vi "System Mixed Checkbox.vi"() -> ()   [LabVIEW 2023]
doc: "Demonstrates how to use the system mixed checkbox."
panel:
  in  "Fail":string="Fail"
  in  "Pass":string="Pass"
  in  "Stop":bool
  in  "Test Result":enum8{"False", "True", "Mixed"}(c332)
  in  "Result List":i32[](listbox)
  # "Overview: Demonstrates the use of the System Mixed Checkbox control.\nInstructions:\n1. Run the VI.\n2. Select an item in the list, and notice its 'Result' value is reflected in the Passed? checkbox.\n3. Select multiple items in the list by Ctrl-clicking on them. If you selected any items with different 'Result' values, the Passed? checkbox will be in a mixed state.\n4. Change the Passed? checkbox value to apply the value to the selected list items.\n5. Click Stop to stop the VI."
  # "For this example, the Allow Mixed option in the System Mixed Checkbox right-click menu is deselected so the user cannot interactively set the checkbox value to a mixed state."
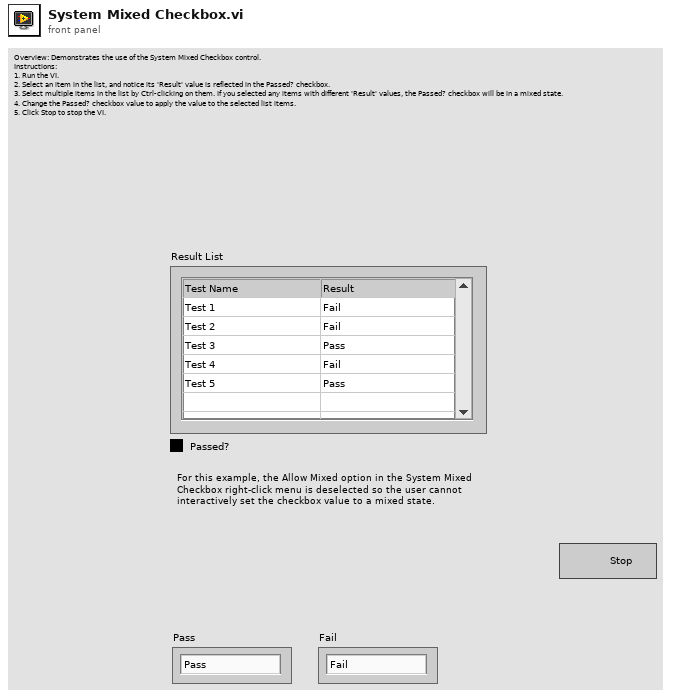
[diagram p1: front panel]
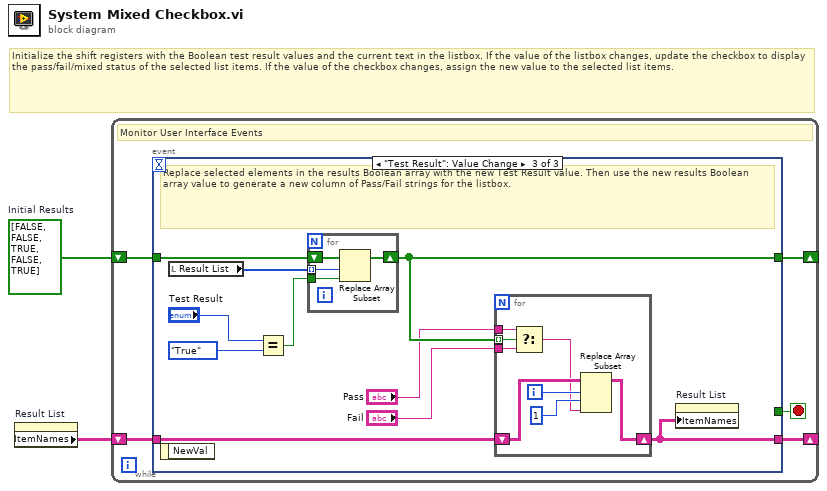
[diagram p0: block diagram]
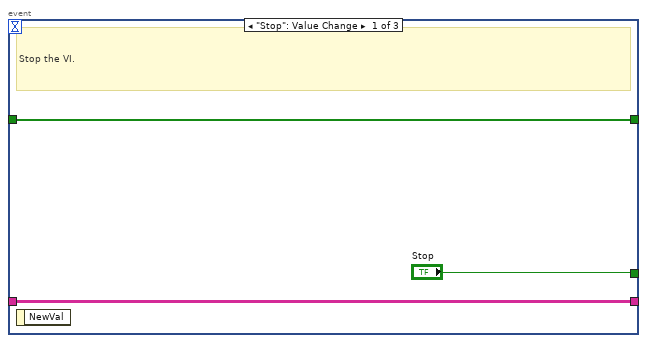
[diagram p2: hidden frame]
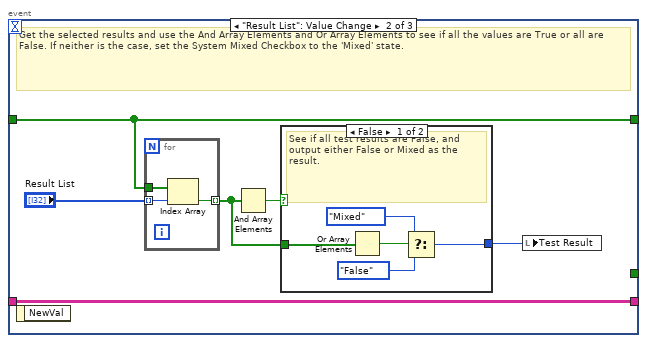
[diagram p3: hidden frame]
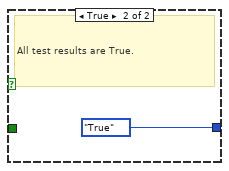
[diagram p4: hidden frame]
diagram:
  w2 = bool[] [FALSE, FALSE, TRUE, FALSE, TRUE]  # Initial Results
  # "Initialize the shift registers with the Boolean test result values and the current text in the listbox. If the value of the listbox changes, update the checkbox to display the pass/fail/mixed status of the selected list items. If the value of the checkbox changes, assign the new value to the selected list items."
  n1 = property on="Result List" class="MCListbox (strict)"() -> ("ItemNames"=w1:string[][])  [unwired: 2 in, 2 out]
  n2 = while {
    shift-right: [w5] -> _
    shift-left: w2 -> [w7]
    shift-right: [w3] -> _
    shift-left: w1 -> [w4]
    stop <- w6 stop-if-true
    # "Monitor User Interface Events"
    n3 = event shown="[2] \"Test Result\": Value Change" {
      selector: _ -> [_ _ _]
      dyn-events: _ -> [_ _ _]
      timeout: _ -> [_ _ _]
      tunnel: w7 -> [w10 w15 w35]
      tunnel: [w10 w15 w32] -> w5
      tunnel: ["Stop" _ _] -> w6
      tunnel: w4 -> [w8 w11 w29]
      tunnel: [w8 w11 w28] -> w3
      event "Stop": Value Change {
        # "Stop the VI."
        n4 = event-data() -> ()  [unwired: 1 in, 1 out]
      }
      event "Result List": Value Change {
        # "Get the selected results and use the And Array Elements and Or Array Elements to see if all the values are True or all are False. If neither is the case, set the System Mixed Checkbox to the 'Mixed' state."
        n5 = event-data() -> ()  [unwired: 1 in, 1 out]
        n6 = for {
          tunnel: "Result List" -> [w25] mode=indexing
          tunnel: w15 -> [w23]
          tunnel: [w24] -> w13 mode=indexing
          n7 = Index Array(array=w23, index=w25) -> (element=w24:bool)
        }
        n8 = And Array Elements(Boolean array=w13) -> (logical AND=w16:bool)
        n9 = case shown="False" w16 {
          tunnel: w13 -> [w18 _]
          tunnel: [w17 enum8{"False", "True", "Mixed"}."True" ("Test Result")] -> w14
          frame False {
            # "See if all test results are False, and output either False or Mixed as the result."
            n10 = Or Array Elements(Boolean array=w18) -> (logical OR=w19:bool)
            n11 = Select(t=enum8{"False", "True", "Mixed"}."Mixed" ("Test Result"), s=w19, f=enum8{"False", "True", "Mixed"}."False" ("Test Result")) -> (s? t:f=w17:enum8{"False", "True", "Mixed"})
          }
          frame True {
            # "All test results are True."
          }
        }
        n12 = local write "Test Result"(w14) -> ()
      }
      event "Test Result": Value Change {
        # "Replace selected elements in the results Boolean array with the new Test Result value. Then use the new results Boolean array value to generate a new column of Pass/Fail strings for the listbox."
        n13 = event-data() -> ()  [unwired: 1 in, 1 out]
        n14 = local read "Result List"() -> (w31:i32[])
        n15 = Equal?(x="Test Result", y=enum8{"False", "True", "Mixed"}."True") -> (x = y?=w33:bool)
        n16 = for {
          tunnel: w31 -> [w47] mode=indexing
          shift-right: [w44] -> w32
          shift-left: w35 -> [w46]
          tunnel: w33 -> [w45]
          n17 = Replace Array Subset(array=w46, new element=w45, index=w47) -> (w44:bool[])
        }
        n18 = for {
          shift-right: [w42] -> w28
          shift-left: w29 -> [w41]
          tunnel: w32 -> [w39] mode=indexing
          tunnel: "Pass" -> [w37]
          tunnel: "Fail" -> [w36]
          i -> [w40]
          n19 = Select(t=w37, s=w39, f=w36) -> (s? t:f=w38:string)
          n20 = Replace Array Subset(array=w41, new element=w38, index (row)=w40, index (col)=1 ("disabled index (col)")) -> (w42:string[][])
        }
        n21 = property on="Result List" class="MCListbox (strict)"("ItemNames"=w28) -> ()  [unwired: 2 in, 2 out]
      }
    }
  }
